vi "Get Bit Depth.vi"(10 "depth":i32, 11 "channel":i32) -> (2 "depth out":i32, 3 "function return":u32)   [LabVIEW 2018, in "Copy of Andor SDK.lvlib"]
doc: "EXPNETTYPE unsigned int WINAPI GetBitDepth(int channel, int * depth);"
uses:
  Copy of Andor SDK.lvlib
  <userlib>/Andor SDK/ATMCD32D.dll
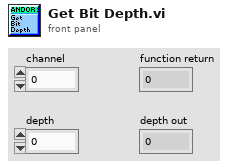
[diagram p1: front panel]
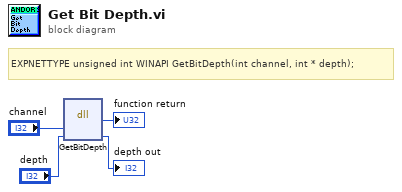
[diagram p0: block diagram]
diagram:
  # "EXPNETTYPE unsigned int WINAPI GetBitDepth(int channel, int * depth);"
  n1 = dll-call lib="C:/Program Files (x86)/National Instruments/LabVIEW 2018/user.lib/Andor SDK/ATMCD32D.*" fn="GetBitDepth"("channel"="channel", "depth"="depth") -> (→"function return":u32, "depth"=→"depth out":i32)  [unwired: 4 in, 2 out]
